vi "VISA RECIVER.vi"() -> ()   [LabVIEW 2017]
uses:
  ad243bfc-ce27-46f1-a81d-b9ecc6892535.vi
  <vilib>/Instr/_visa.llb/VISA Configure Serial Port (Instr).vi
panel:
  out "error out":errorcluster
  out "read buffer":string
  in  "timeout (10sec)":u32=2000
  in  "Enable Termination Char (T)":bool
  in  "baud rate":u32=9600
  in  "VISA resource name":refnum<visa-resource-name>
  in  "stop":bool
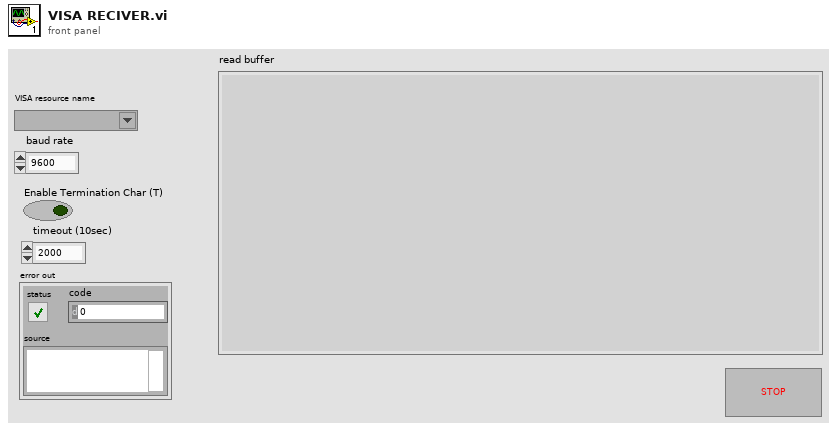
[diagram p1: front panel]
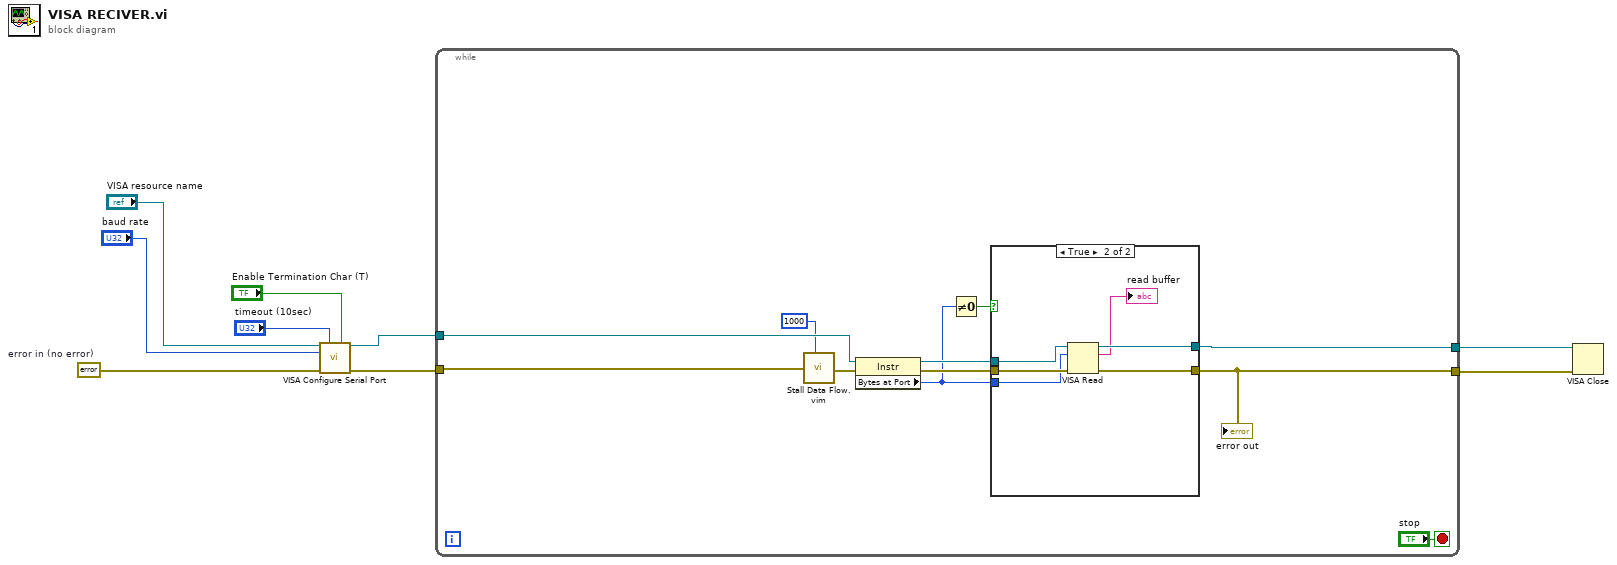
[diagram p0: block diagram]
diagram:
  w4 = errorcluster {"status"=FALSE, "code"=0, "source"=""}  # error in (no error)
  n1 = call-poly "VISA Configure Serial Port"("VISA resource name"="VISA resource name", "timeout (10sec)"="timeout (10sec)", "Enable Termination\nChar (T)"="Enable Termination Char (T)", "baud rate (9600)"="baud rate", "error in (no error)"=w4) -> ("VISA resource name out"=w2:refnum<visa-resource-name>, "error out"=w5:errorcluster)  [unwired: 9 in]
  n2 = while {
    tunnel: w5 -> [w13]
    tunnel: [w15] -> w6
    tunnel: w2 -> [w17]
    tunnel: [w16] -> w1
    stop <- "stop" stop-if-true
    n3 = call "Stall Data Flow.vim"("value in"=w13, "milliseconds to wait"=1000) -> ("value out"=w14:errorcluster)  [unwired: 1 out]
    n4 = property class="Instr"(reference=w17, error in=w14) -> (reference out=w18:refnum<visa-resource-name>, error out=w19:errorcluster, "Bytes at Port"=w10:u32)
    n5 = Not Equal To 0?(x=w10) -> (x != 0?=w11:bool)
    n6 = case shown="True" w11 {
      tunnel: w19 -> [w22 w28]
      tunnel: w18 -> [w21 w27]
      tunnel: w10 -> [_ w26]
      tunnel: [w21 w25] -> w16
      tunnel: [w22 w24] -> w15
      frame False {
      }
      frame True {
        n7 = VISA Read(VISA resource name=w27, byte count=w26, error in (no error)=w28) -> (VISA resource name out=w25:refnum<visa-resource-name>, read buffer=→"read buffer":string, error out=w24:errorcluster)  [unwired: 1 out]
      }
    }
    "error out" <- w15
  }
  n8 = VISA Close(VISA resource name=w1, error in (no error)=w6) -> ()  [unwired: 1 out]
